vi "UDCStart.vi"(8 "Error In":errorcluster, 9 "configString":string, 10 "locationID":string, 11 "clientID":string) -> (0 "Error Out":errorcluster)   [LabVIEW 2020, in "niceiplib.lvlib"]
doc: "This API is used to start the UDC. It is advised to call this API in the place where the initialization of the Application is done."
uses:
  <vilib>/UDC/niceiplib.lvlib
panel:
  # "@param[in]\tclientID    \t\nYour <a href=\"http://niweb.natinst.com/confluence/display/UDC/UDC+FAQ#UDCFAQ-Whatistheproductid%3FHowwillIdecideit%3F\">client ID</a>\n @param[in]\tlocationID  \t\nThis is the locationID for your product. See @ref location\n @param[in]\tconfigString\t\nThis is for further session level configurations @ref configString"
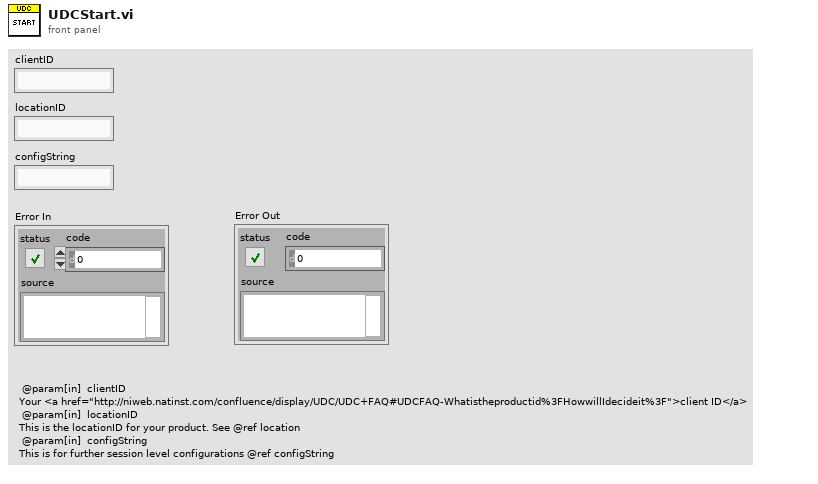
[diagram p1: front panel]
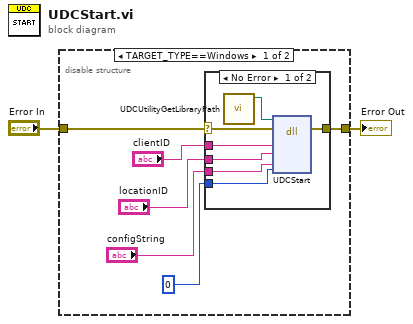
[diagram p0: block diagram]
diagram:
  n1 = disable-structure shown="TARGET_TYPE==Windows" {
    disable-tunnel: [w4 w17] -> w2
    disable-tunnel: "Error In" -> [w3 w17]
    frame condition #0 (active) {
      n2 = case shown="No Error" w3 {
        selector: w3 -> [w10 w16]
        tunnel: "clientID" -> [w15 _]
        tunnel: "locationID" -> [w14 _]
        tunnel: "configString" -> [w13 _]
        tunnel: 0 ("uploadProcess") -> [w12 _]
        tunnel: [w11 w16] -> w4
        frame No Error {
          n3 = call <vilib>:"UDCUtilityGetLibraryPath.vi"() -> ("Library Path"=w9:path)  [unwired: 11 in]
          n4 = dll-call lib="C:/2013LabVIEWCode/dist/vi.lib/UDC/niceiplib.*" fn="UDCStart"(path in=w9, error in=w10, "clientID"=w15, "locationID"=w14, "configString"=w13, "uploadProcess"=w12) -> (error out=w11:errorcluster)  [unwired: 6 in, 1 out]
        }
        frame Error {
        }
      }
    }
    frame condition #1 {
    }
  }
  "Error Out" <- w2
